vi "Insert Line Into File.vi"(7 "Check Only? (f)":bool, 8 "Error In":errorcluster, 9 "Line":string="i2c-bcm2708", 10 "File Path":string="cat /etc/modules", 11 "Install LV Data":T1={"SSH Session"=refnum, "Status Log"="", "Detailed Log"="", "Credentials"={"Hostname or IP"="192.168.7.2", "Username"="root", "Password"=""}, "Target Info"={"OS Version"="", "CPU"="", "Systemd Version"="", "Internet Access"=FALSE, "Device Type"="", "LV Installed Ver"="", "LV Available Ver"="", "LV Upgrade Available"=FALSE, "Hostname"="", "NIC Info"=[]}, "Reboot Required?"=FALSE}) -> (0 "Error Out":errorcluster, 1 "Log":string, 2 "Line Alredy Present?":bool, 3 "Install LV Data":T1={"SSH Session"=refnum, "Status Log"="", "Detailed Log"="", "Credentials"={"Hostname or IP"="192.168.7.2", "Username"="root", "Password"=""}, "Target Info"={"OS Version"="", "CPU"="", "Systemd Version"="", "Internet Access"=FALSE, "Device Type"="", "LV Installed Ver"="", "LV Available Ver"="", "LV Upgrade Available"=FALSE, "Hostname"="", "NIC Info"=[]}, "Reboot Required?"=FALSE})   [LabVIEW 2019, in "LMH-LINX.lvlib"]
uses:
  <vilib>/MakerHub/LINX/LMH-LINX.lvlib
  <vilib>/MakerHub/LINX/Private/Utilties/Target Management/Install LV Data.ctl
  E:/lv2019/dist/vi.lib/MakerHub/LINX/Resources/Renci.SshNet.dll
  Resources/Renci.SshNet.dll
  <vilib>/MakerHub/LINX/Private/Utilties/Target Management/Target Info.ctl
  <vilib>/MakerHub/LINX/Private/Utilties/Target Management/NIC Info.ctl
  <vilib>/MakerHub/LINX/Private/Utilties/Target Management/NIC Mode.ctl
  <vilib>/regexp/Match Regular Expression.xnode
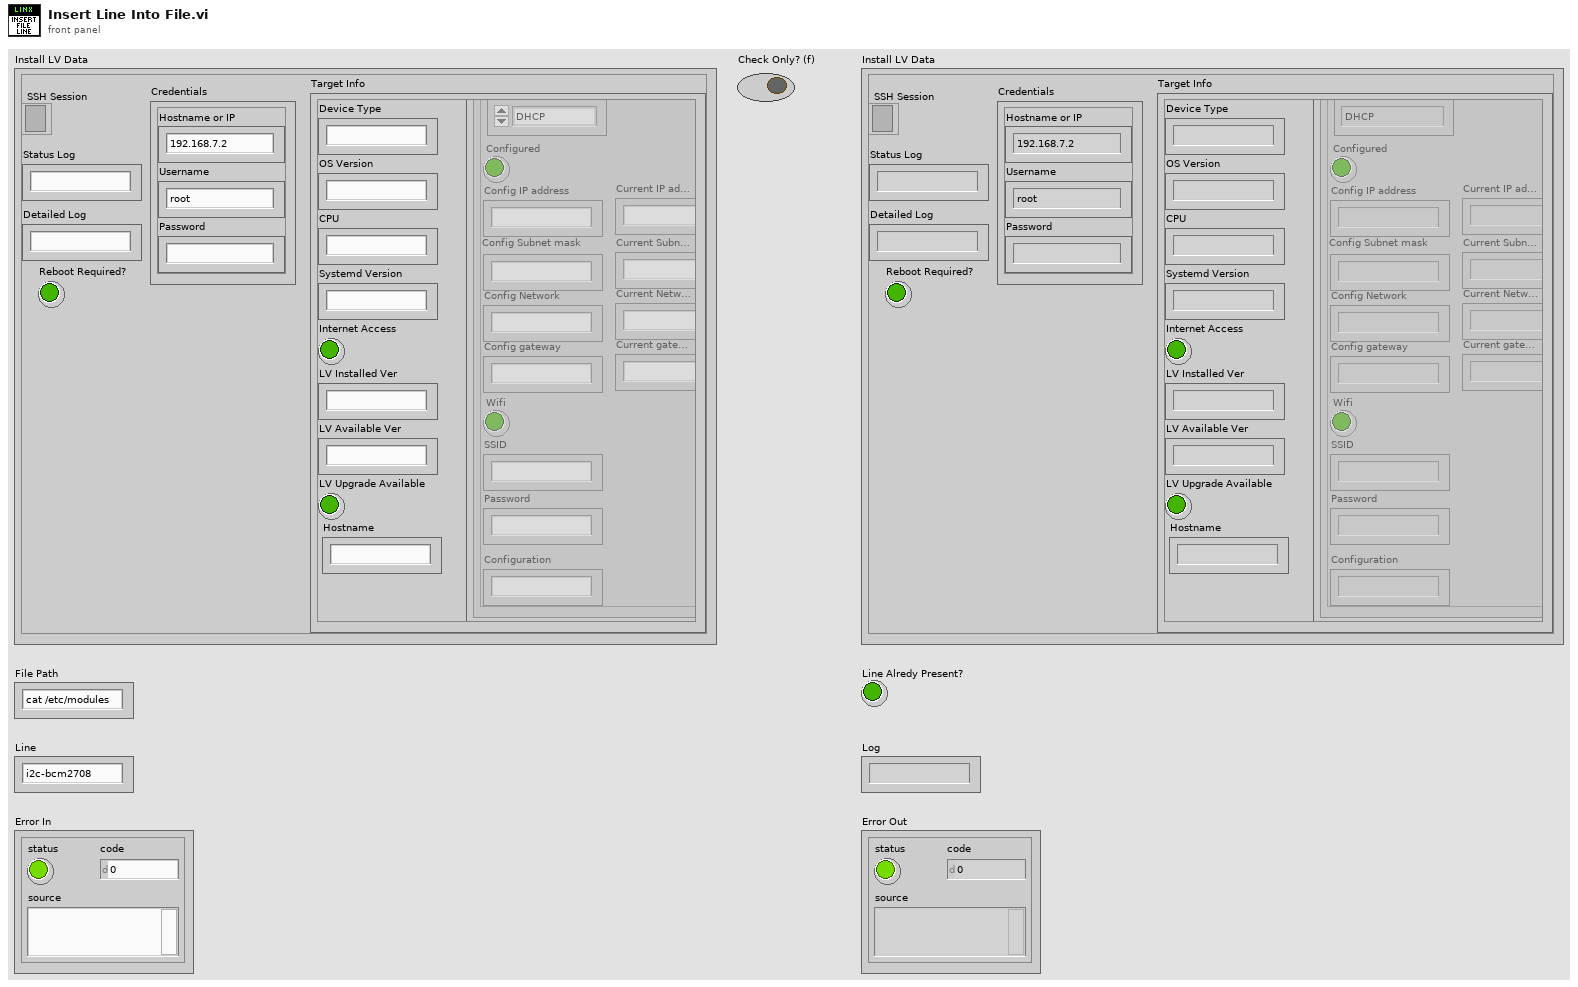
[diagram p1: front panel]
types:
  T1 = typedef "LMH-LINX.lvlib/Install LV Data.ctl" = cluster{"SSH Session":refnum<k24>, "Status Log":string, "Detailed Log":string, "Credentials":cluster{"Hostname or IP":string, "Username":string, "Password":string}, "Target Info":T2, "Reboot Required?":bool}
  T2 = typedef "LMH-LINX.lvlib/Target Info.ctl" = cluster{"OS Version":string, "CPU":string, "Systemd Version":string, "Internet Access":bool, "Device Type":string, "LV Installed Ver":string, "LV Available Ver":string, "LV Upgrade Available":bool, "Hostname":string, "NIC Info":T3[]}
  T3 = typedef "LMH-LINX.lvlib/NIC Info.ctl" = cluster{"Name":string, "NIC Mode":T4, "Configured":bool, "Config IP address":string, "Config Subnet mask":string, "Config Network":string, "Config gateway":string, "Wifi":bool, "SSID":string, "Password":string, "Configuration":string, "Current IP address":string, "Current Subnet mask":string, "Current gateway":string, "Current Network":string}
  T4 = typedef "LMH-LINX.lvlib/NIC Mode.ctl" = enum16{"DHCP", "Static", "Loopback"}
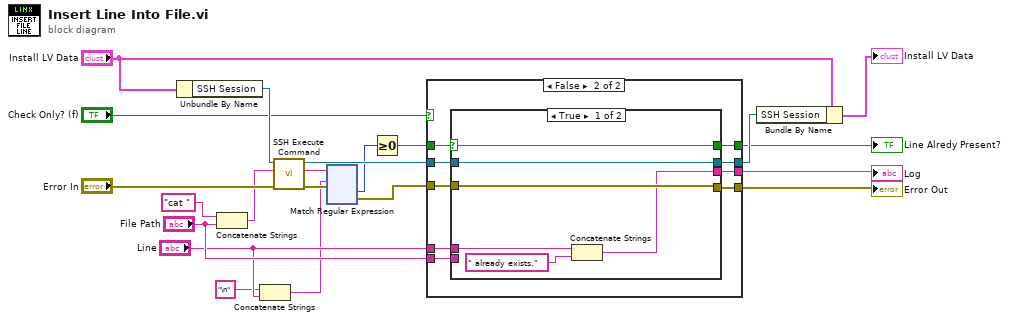
[diagram p0: block diagram]
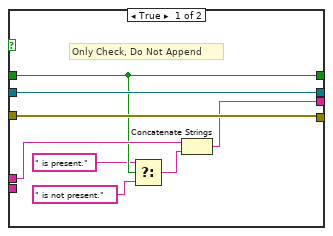
[diagram p2: hidden frame]
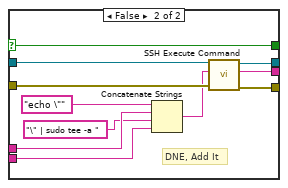
[diagram p3: hidden frame]
diagram:
  n1 = Unbundle By Name("Install LV Data") -> ("SSH Session"=w19:refnum<k24>)
  n2 = Concatenate Strings("cat " ("string"), "File Path") -> (w10:string)
  n3 = Concatenate Strings("\n", "Line") -> (w2:string)
  n4 = call <vilib>:"SSH Execute Command.vi"("Error In"="Error In", "Command"=w10, "SSH Session"=w19) -> ("Error Out"=w16:errorcluster, "Std Out"=w12:string, "SSH Session"=w17:refnum<k24>)  [unwired: 6 in]
  n5 = xnode "Match Regular Expression"("input string"=w12, "regular expression"=w2, "error in"=w16) -> ("offset past match"=w14:i32, "error out"=w15:errorcluster)  [unwired: 3 in, 3 out]
  n6 = Greater Or Equal To 0?(x=w14) -> (x >= 0?=w13:bool)
  n7 = case shown="False" "Check Only? (f)" {
    tunnel: w17 -> [w29 w38]
    tunnel: w15 -> [w28 w37]
    tunnel: w13 -> [w25 w36]
    tunnel: "Line" -> [w26 w35]
    tunnel: [w28 w34] -> w9
    tunnel: [w27 w33] -> w8
    tunnel: [w29 w32] -> w7
    tunnel: "File Path" -> [_ w31]
    tunnel: [w25 w30] -> w4
    frame True {
      # "Only Check, Do Not Append"
      n8 = Select(t=" is present.", s=w25, f=" is not present.") -> (s? t:f=w22:string)
      n9 = Concatenate Strings(w26, w22) -> (w27:string)
    }
    frame False {
      n10 = case shown="True" w36 {
        selector: w36 -> [w39 w45]
        tunnel: [w40 w55] -> w33
        tunnel: [w44 w54] -> w34
        tunnel: [w43 w53] -> w32
        tunnel: w38 -> [w43 w52]
        tunnel: w37 -> [w44 w51]
        tunnel: w35 -> [w42 w49]
        tunnel: w31 -> [_ w47]
        tunnel: [w39 w45] -> w30
        frame True {
          n11 = Concatenate Strings(w42, " already exists." ("Std Out")) -> (w40:string)
        }
        frame False {
          # "DNE, Add It"
          n12 = Concatenate Strings("echo \"", w49, "\" | sudo tee -a " ("string"), w47) -> (w46:string)
          n13 = call <vilib>:"SSH Execute Command.vi"("Error In"=w51, "Command"=w46, "SSH Session"=w52) -> ("Error Out"=w54:errorcluster, "Std Out"=w55:string, "SSH Session"=w53:refnum<k24>)  [unwired: 6 in]
        }
      }
    }
  }
  "Log" <- w8
  "Error Out" <- w9
  "Line Alredy Present?" <- w4
  n14 = Bundle By Name(cluster="Install LV Data", "SSH Session"=w7) -> (→"Install LV Data":T1)
